vi "Global 2.vi"() -> ()   [LabVIEW 2016]
panel:
  in  "Gyro":dbl
  in  "Shooter Velocity":dbl
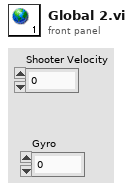
[diagram p1: front panel]
diagram:
